vi "Flow Rate.vi"() -> ()   [LabVIEW 2018]
panel:
  out "Flow Rate (kg/min)":dbl
  in  "AveA1":dbl
  in  "EE1":dbl
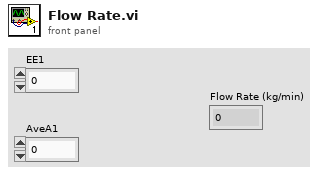
[diagram p1: front panel]
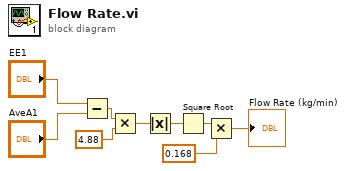
[diagram p0: block diagram]
diagram:
  n1 = Subtract(x="EE1", y="AveA1") -> (x-y=w6:dbl)
  n2 = Multiply(x=w6, y=4.88) -> (x*y=w4:dbl)
  n3 = Absolute Value(x=w4) -> (abs(x)=w7:dbl)
  n4 = Square Root(x=w7) -> (sqrt(x)=w3:dbl)
  n5 = Multiply(x=w3, y=0.168) -> (x*y=→"Flow Rate (kg/min)":dbl)
